vi "gridfruit pi side mk2 (1).vi"() -> ()   [LabVIEW 2020]
doc: "This VI implements a client for the TCP Named Service - Server.vi. It connects to a service by specifying the server address and the name of the service. The client receives the string sent by the server, displays the string and closes the connection."
panel:
  in  "Status file":path=path "/home/pi/Documents/Driver Code/dummy.txt"
  out "system readouts":T1
  in  "Driver status file":path=path "/home/pi/Documents/Driver Code/Driver Status.txt"
  # "Overview: Demonstrates the use of the TCP functions to connect to a TCP server VI via named service and receive data.\nInstructions:\n1. Ensure TCP Named Service - Server.vi is already running.\n2. Run the VI."
  # "ADR enabled"
  # "Pre-cooling start time"
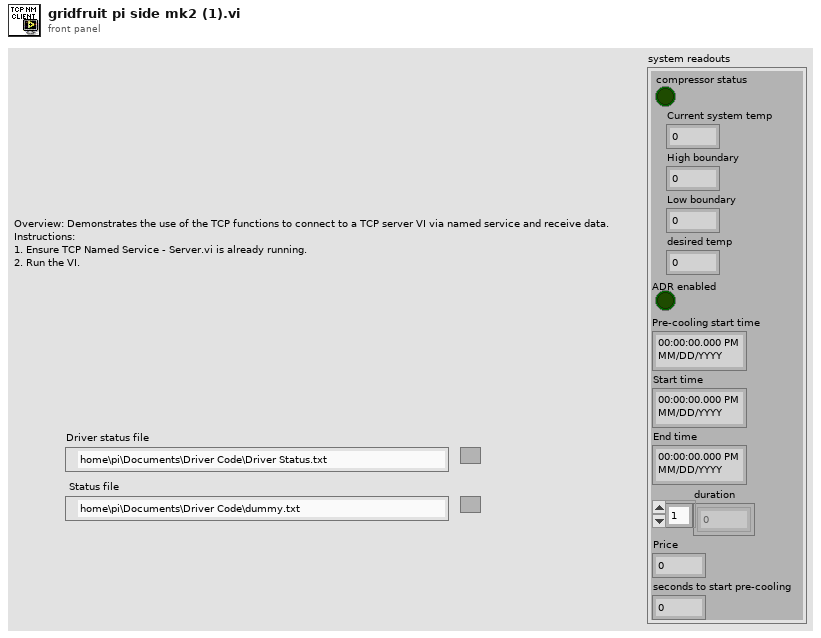
[diagram p1: front panel]
types:
  T1 = cluster{"compressor status":bool, "Current system temp":dbl, "High boundary":dbl, "Low boundary":dbl, "desired temp":dbl, bool, timestamp, "Start time":timestamp, "End time":timestamp, "duration":dbl[], "Price":dbl, "seconds to start pre-cooling":dbl}
  T2 = cluster{"compressor status":bool, "Current system temp":dbl, "High boundary":dbl, "Low boundary":dbl, "Desired temp":dbl, "ADR enabled":bool, "Pre-cooling start":timestamp, "Start time":timestamp, "End time":timestamp, "duration":dbl[], "Price":dbl, "pre-cooling seconds":dbl}
  T3 = enum16{"open", "replace", "create", "open or create", "replace or create", "replace or create with confirmation"}
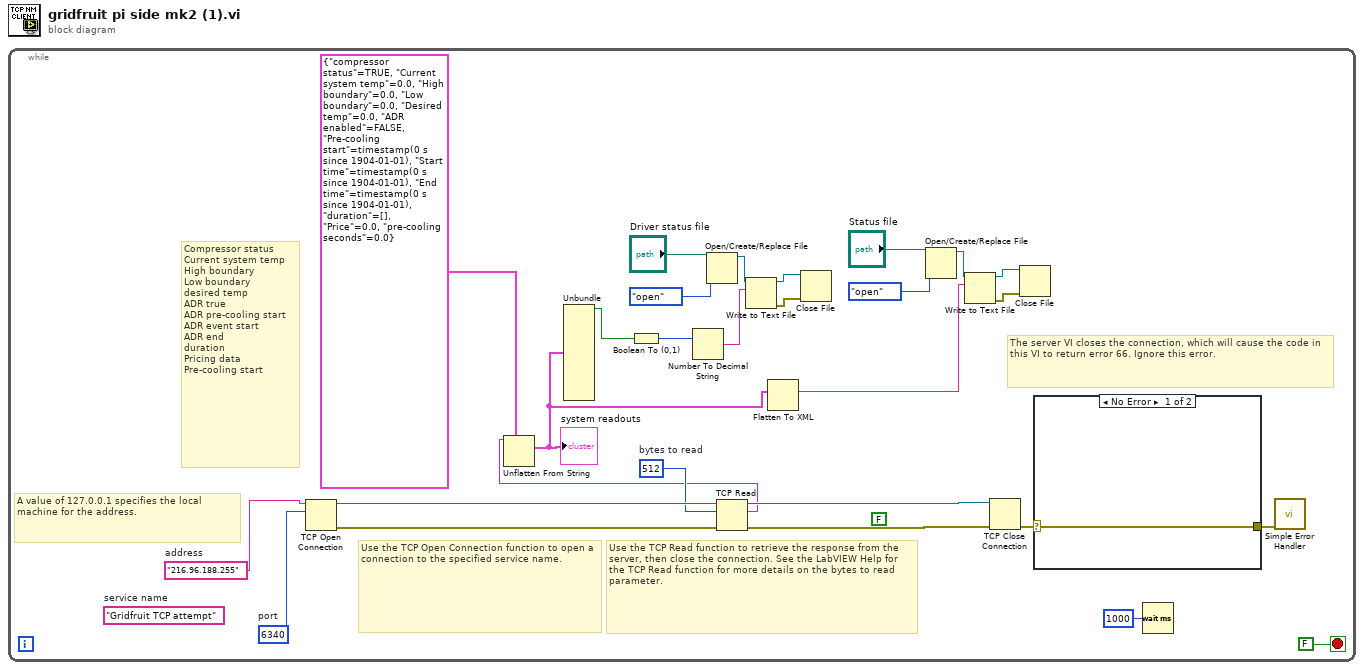
[diagram p0: block diagram]
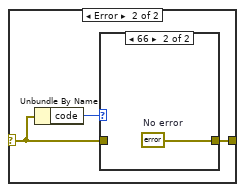
[diagram p2: hidden frame]
diagram:
  n1 = while {
    stop <- FALSE stop-if-true
    (unwired) FALSE
    w15 = 512  # bytes to read
    w21 = u16 6340  # port
    (unwired) "Gridfruit TCP attempt"  # service name
    w22 = "216.96.188.255"  # address
    # "Compressor status\nCurrent system temp\nHigh boundary\nLow boundary\ndesired temp\nADR true\nADR pre-cooling start\nADR event start\nADR end\nduration\nPricing data\nPre-cooling start"
    # "The server VI closes the connection, which will cause the code in this VI to return error 66. Ignore this error."
    # "Use the TCP Open Connection function to open a connection to the specified service name."
    # "Use the TCP Read function to retrieve the response from the server, then close the connection. See the LabVIEW Help for the TCP Read function for more details on the bytes to read parameter."
    # "A value of 127.0.0.1 specifies the local machine for the address."
    n2 = TCP Open Connection(address=w22, remote port or service name=w21) -> (connection ID=w27:refnum<k5>, error out=w28:errorcluster)  [unwired: 3 in]
    n3 = Open/Create/Replace File(file path (use dialog)="Driver status file", operation (0:open)=T3."open") -> (refnum out=w17:refnum<file>)  [unwired: 4 in, 2 out]
    n4 = TCP Read(connection ID=w27, bytes to read=w15, error in (no error)=w28) -> (connection ID out=w26:refnum<k5>, data out=w2:string, error out=w25:errorcluster)  [unwired: 2 in]
    n5 = Unflatten From String(type=T2 {"compressor status"=TRUE, "Current system temp"=0.0, "High boundary"=0.0, "Low boundary"=0.0, "Desired temp"=0.0, "ADR enabled"=FALSE, "Pre-cooling start"=timestamp(0 s since 1904-01-01), "Start time"=timestamp(0 s since 1904-01-01), "End time"=timestamp(0 s since 1904-01-01), "duration"=[], "Price"=0.0, "pre-cooling seconds"=0.0} ("output cluster"), binary string=w2) -> (value=w9:T2)  [unwired: 3 in, 2 out]
    "system readouts" <- w9
    n6 = Unbundle(w9) -> ("compressor status"=w12:bool)  [unwired: 11 out]
    n7 = Boolean To (0,1)(Boolean=w12) -> (0, 1=w11:i16)
    n8 = Number To Decimal String(number=w11) -> (decimal integer string=w10:string)  [unwired: 1 in]
    n9 = Write to Text File(file (use dialog)=w17, text=w10) -> (refnum out=w20:refnum<file>, error out=w19:errorcluster)  [unwired: 2 in, 1 out]
    n10 = Flatten To XML(6:w9) -> (2:w1:string)
    n11 = Close File(refnum=w20, error in=w19) -> ()  [unwired: 2 out]
    n12 = Open/Create/Replace File(file path (use dialog)="Status file", operation (0:open)=T3."open") -> (refnum out=w5:refnum<file>)  [unwired: 4 in, 2 out]
    n13 = Write to Text File(file (use dialog)=w5, text=w1) -> (refnum out=w8:refnum<file>, error out=w7:errorcluster)  [unwired: 2 in, 1 out]
    n14 = TCP Close Connection(connection ID=w26, error in (no error)=w25) -> (error out=w24:errorcluster)  [unwired: 1 in, 1 out]
    n15 = Close File(refnum=w8, error in=w7) -> ()  [unwired: 2 out]
    n16 = case shown="No Error" w24 {
      selector: w24 -> [w29 w31]
      tunnel: [w29 w30] -> w23
      frame No Error {
      }
      frame Error {
        n17 = Unbundle By Name(w31) -> ("code"=w32:i32)
        n18 = case shown="66" w32 {
          tunnel: w31 -> [w33 _]
          tunnel: [w33 w34] -> w30
          frame Default {
          }
          frame 66 {
            w34 = errorcluster {"status"=FALSE, "code"=0, "source"=""}  # No error
          }
        }
      }
    }
    n19 = Wait (ms)(milliseconds to wait=u32 1000) -> ()  [unwired: 1 out]
    n20 = call <vilib>:"Simple Error Handler.vi"("error in (no error)"=w23) -> ()  [unwired: 4 in, 5 out]
  }
